vi "ParametersUpdated.vi"(8 "error in (no error)":errorcluster, 10 "Current Parameters":T1, 11 "SpectrometerUI in":refnum<class "SpectrometerUI.lvclass">) -> (0 "error out":errorcluster, 3 "SpectrometerUI out":refnum<class "SpectrometerUI.lvclass">)   [LabVIEW 2023, in "SpectrometerUI.lvlib" / "SpectrometerUI.lvclass"]
uses:
  SpectrometerUI.lvclass
  SpectrometerUI.lvclass/SpectrometerUI.ctl
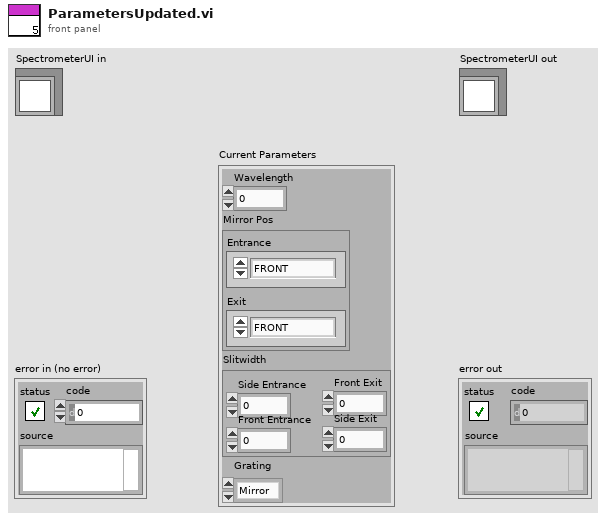
[diagram p1: front panel]
types:
  T1 = cluster{"Wavelength":dbl, "Mirror Pos":cluster{"Entrance":enum16{"FRONT", "SIDE"}, "Exit":enum16{"FRONT", "SIDE"}}, "Slitwidth":cluster{"Side Entrance":u16, "Front Entrance":u16, "Front Exit":u16, "Side Exit":u16}, "Grating":enum16{"Mirror", "1200 g/mm", "1800 g/mm"}}
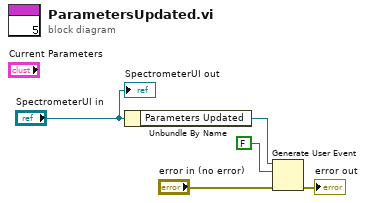
[diagram p0: block diagram]
diagram:
  n1 = Unbundle By Name("SpectrometerUI in") -> ("Parameters Updated"=w4:refnum<user-event>)
  n2 = Generate User Event(user event=w4, event data cluster=FALSE ("event data"), error in="error in (no error)") -> (error out=→"error out":errorcluster)  [unwired: 1 in, 1 out]
  "SpectrometerUI out" <- "SpectrometerUI in"
